vi "PM-P-distribute_data.vi"(8 "error in (no error)":errorcluster, 11 "loop data":T1) -> (0 "error out":errorcluster, 3 "loop data":T1)   [LabVIEW 2018]
uses:
  PM-P-loop_data.ctl
  PM-P-user_events.ctl
  init-close/PM-common-heartrate_data.ctl
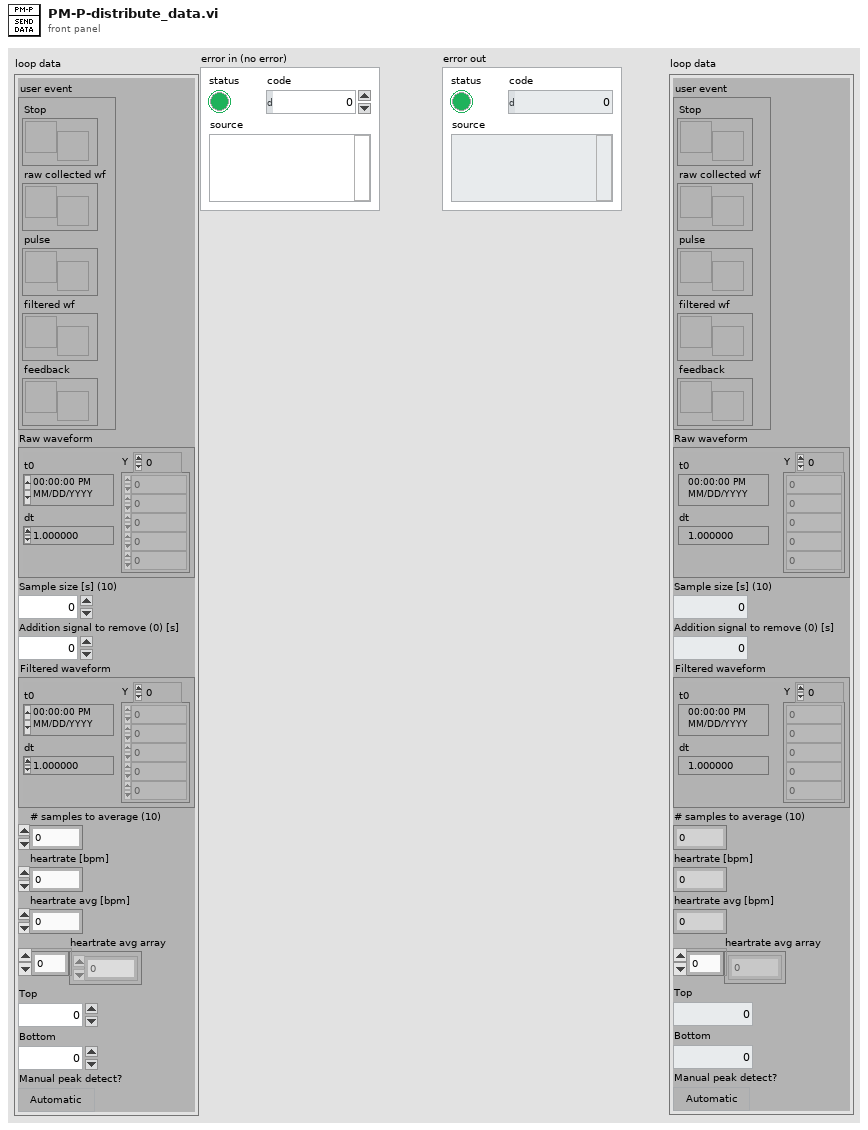
[diagram p1: front panel]
types:
  T1 = typedef "PM-P-loop_data.ctl" = cluster{"user event":T2, "Raw waveform":waveform(dbl), "Sample size [s] (10)":i32, "Addition signal to remove (0) [s]":dbl, "Filtered waveform":waveform(dbl), "# samples to average (10)":i32, "heartrate [bpm]":dbl, "heartrate avg [bpm]":dbl, "heartrate avg array":dbl[], "Top":dbl, "Bottom":dbl, "Manual peak detect?":bool}
  T2 = typedef "PM-P-user_events.ctl" = cluster{"Stop":refnum<user-event>, "raw collected wf":refnum<user-event>, "pulse":refnum<user-event>, "filtered wf":refnum<user-event>, "feedback":refnum<user-event>}
  T3 = typedef "PM-common-heartrate_data.ctl" = cluster{"heartrate":dbl, "heartrate avg":dbl}
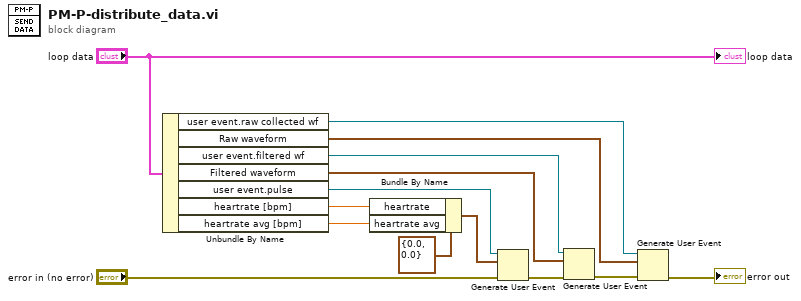
[diagram p0: block diagram]
diagram:
  n1 = Unbundle By Name("loop data") -> ("user event.raw collected wf"=w2:refnum<user-event>, "Raw waveform"=w1:waveform(dbl), "user event.filtered wf"=w4:refnum<user-event>, "Filtered waveform"=w3:waveform(dbl), "user event.pulse"=w9:refnum<user-event>, "heartrate [bpm]"=w6:dbl, "heartrate avg [bpm]"=w5:dbl)
  n2 = Bundle By Name(cluster=T3 {"heartrate"=0.0, "heartrate avg"=0.0} ("event data"), "heartrate"=w6, "heartrate avg"=w5) -> (w7:T3)
  n3 = Generate User Event(user event=w9, event data cluster=w7, error in="error in (no error)") -> (error out=w13:errorcluster)  [unwired: 1 in, 1 out]
  n4 = Generate User Event(user event=w4, event data cluster=w3, error in=w13) -> (error out=w14:errorcluster)  [unwired: 1 in, 1 out]
  n5 = Generate User Event(user event=w2, event data cluster=w1, error in=w14) -> (error out=→"error out":errorcluster)  [unwired: 1 in, 1 out]
  "loop data" <- "loop data"
